vi "Configure Source.vi"(8 "error in (no error)":errorcluster, 10 "Source (F:Volt)":bool, 11 "E3610x in":refnum<class "E3610x.lvclass">) -> (0 "error out":errorcluster, 3 "E3610x out":refnum<class "E3610x.lvclass">)   [LabVIEW 2020, in "E3610x.lvclass"]
uses:
  E3610x.lvclass
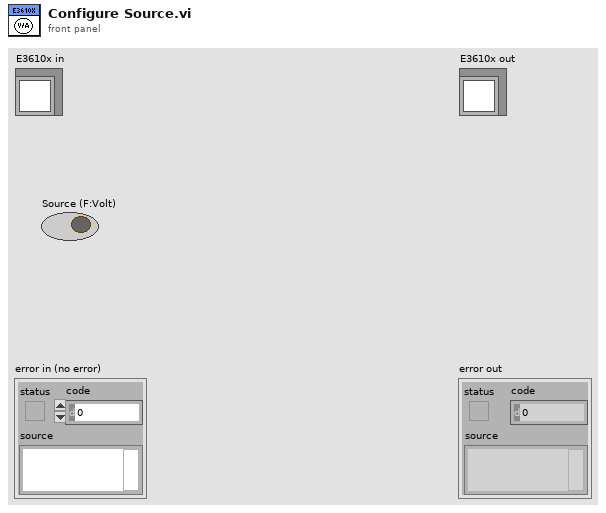
[diagram p1: front panel]
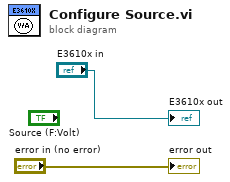
[diagram p0: block diagram]
diagram:
  "error out" <- "error in (no error)"
  "E3610x out" <- "E3610x in"
